vi "open connection.vi"(8 "error in (no error)":errorcluster, 11 "CEG4500 in":refnum<class "CEG4500.lvclass">) -> (0 "error out":errorcluster, 3 "CEG4500 out":refnum<class "CEG4500.lvclass">)   [LabVIEW 2013, in "CEG4500.lvclass"]
uses:
  CEG4500.lvclass
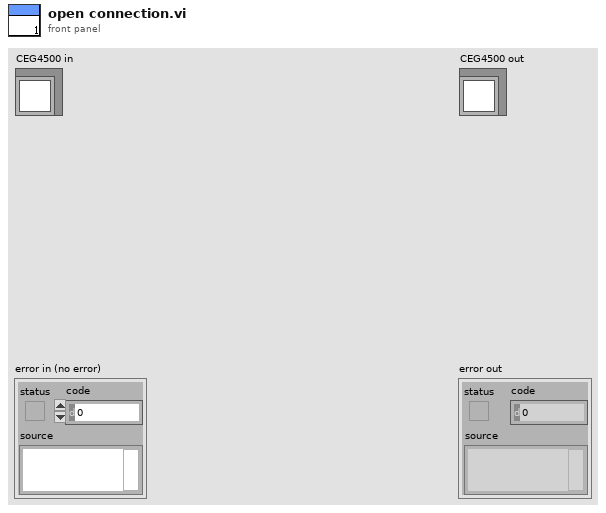
[diagram p1: front panel]
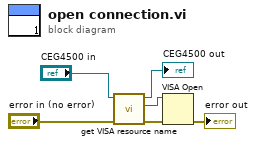
[diagram p0: block diagram]
diagram:
  n1 = call-dynamic "get VISA resource name.vi"("error in (no error)"="error in (no error)", "DeviceInterface (Eingang)"="CEG4500 in") -> ("error out"=w1:errorcluster, "VISA resource name"=w2:refnum<visa-resource-name>, "DeviceInterface (Ausgang)"=→"CEG4500 out":refnum<class "CEG4500.lvclass">)  [unwired: 7 in]
  n2 = VISA Open(error in (no error)=w1, VISA resource name=w2) -> (error out=→"error out":errorcluster)  [unwired: 3 in, 1 out]
